vi "StopTask.vi"(2 "error in (no error)":errorcluster, 3 "StepperController in":refnum<class "StepperController.lvclass">) -> (0 "error out":errorcluster, 1 "StepperController out":refnum<class "StepperController.lvclass">)   [LabVIEW 2013, in "StepperController.lvclass"]
uses:
  StepperController.lvclass
  StepperController.lvclass/StepperController.ctl
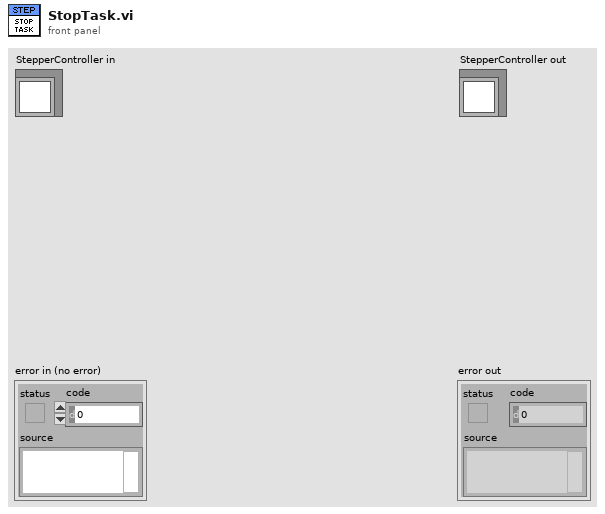
[diagram p1: front panel]
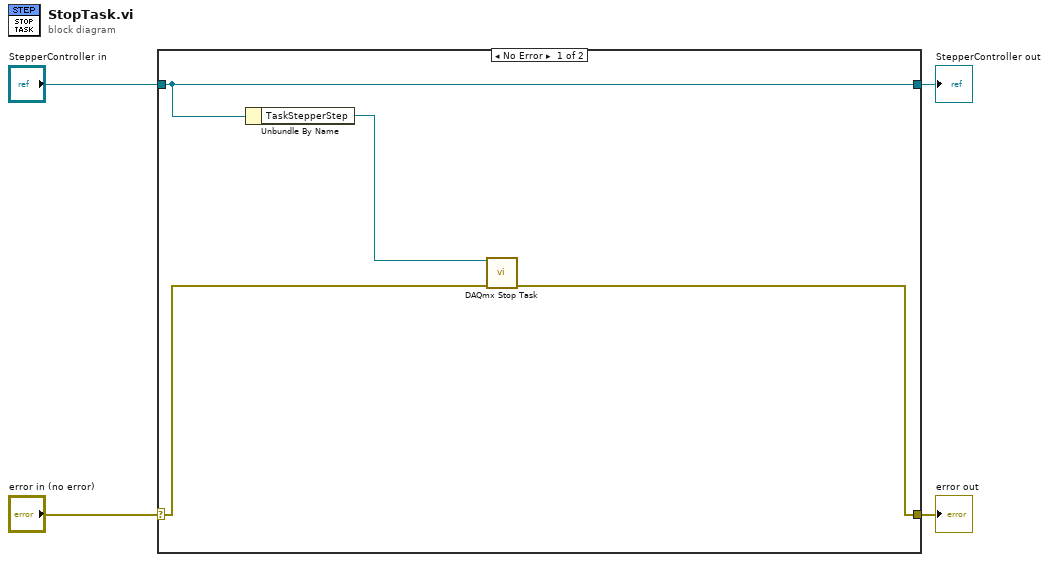
[diagram p0: block diagram]
diagram:
  n1 = case shown="No Error" "error in (no error)" {
    selector: "error in (no error)" -> [w6 w9]
    tunnel: [w5 w9] -> w3
    tunnel: [w8 w10] -> w1
    tunnel: "StepperController in" -> [w8 w10]
    frame No Error {
      n2 = Unbundle By Name(w8) -> ("TaskStepperStep"=w7:refnum<k21>)
      n3 = call <vilib>:"DAQmx Stop Task.vi"("task/channels in"=w7, "error in"=w6) -> ("error out"=w5:errorcluster)  [unwired: 12 in, 1 out]
    }
    frame Error {
    }
  }
  "error out" <- w3
  "StepperController out" <- w1
